vi "contains.vi"(0 "reference":refnum<class "PointNode.lvclass">, 1 "point2D":T1 {"y" format="%.2f"; "x" format="%.2f"}, 2 "AdditionalMargin":i32, 5 "error in (no error)":errorcluster) -> (14 "reference out":refnum<class "PointNode.lvclass">, 15 "contains":bool, 19 "error out":errorcluster)   [LabVIEW 2016, in "PointNode.lvclass"]
doc: "public boolean contains(Point2D p)"
uses:
  <resource>/Framework/Providers/Open_GDS/UML/PointNode_class/PointNode.lvclass
  <resource>/Framework/Providers/Open_GDS/UML/General/Point/Point Point2D.ctl
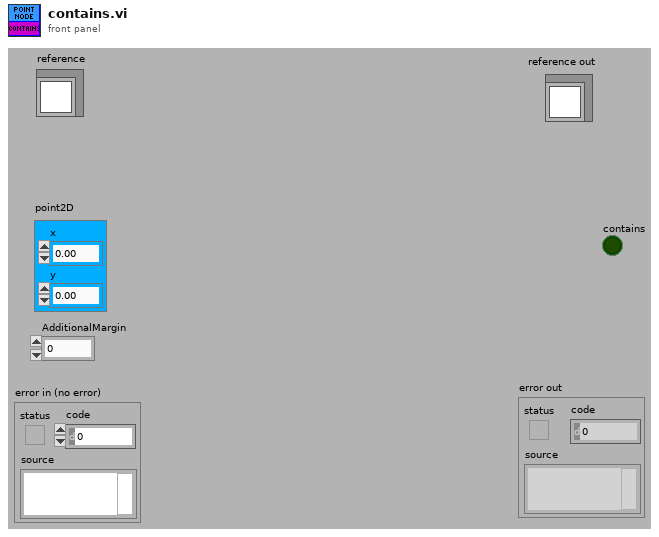
[diagram p1: front panel]
types:
  T1 = typedef "Point Point2D.ctl" = cluster{"x":dbl, "y":dbl}
  T2 = typedef "PointNode.lvclass/ObjectAttributes.ctl" = cluster{"point":T1}
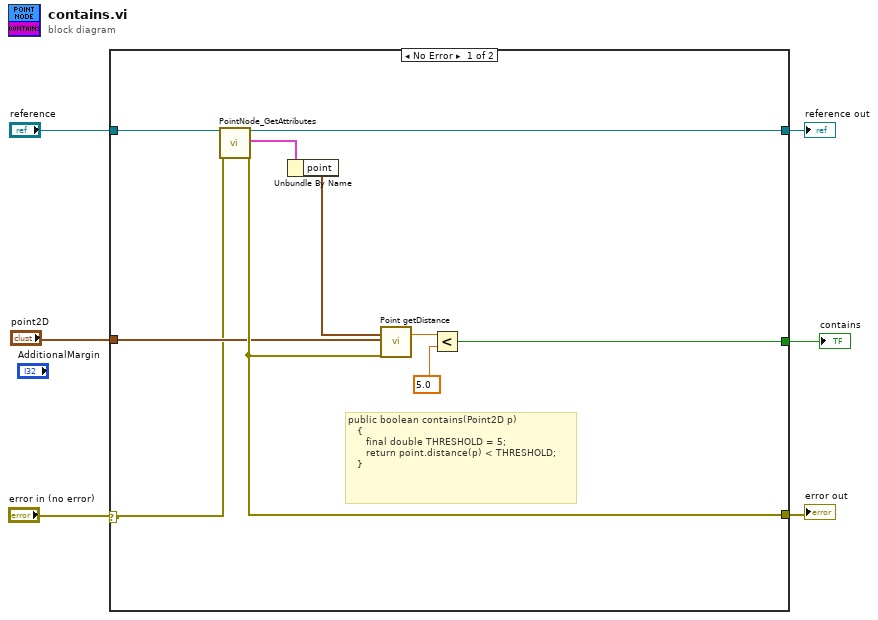
[diagram p0: block diagram]
diagram:
  n1 = case shown="No Error" "error in (no error)" {
    selector: "error in (no error)" -> [w8 w17]
    tunnel: "reference" -> [w16 w18]
    tunnel: [w15 w17] -> w5
    tunnel: [w14 w18] -> w4
    tunnel: "point2D" -> [w13 _]
    tunnel: [w12 _] -> w1
    frame No Error {
      # "public boolean contains(Point2D p)\n   {\n      final double THRESHOLD = 5;\n      return point.distance(p) < THRESHOLD;\n   }"
      n2 = call <resource>:"PointNode_GetAttributes.vi"("reference in"=w16, "error in (no error)"=w8) -> ("reference out"=w14:refnum<class "PointNode.lvclass">, "Data"=w7:T2, "error out"=w15:errorcluster)  [unwired: 1 in, 14 out]
      n3 = Unbundle By Name(w7) -> ("point"=w11:T1)
      n4 = call <resource>:"Point getDistance.vi"("point1"=w11, "point2"=w13, "error in (no error)"=w15) -> ("distance"=w10:dbl)  [unwired: 16 out]
      n5 = Less?(x=w10, y=5.0) -> (x < y?=w12:bool)
    }
    frame Error {
    }
  }
  "reference out" <- w4
  "error out" <- w5
  "contains" <- w1
